vi "Get Wires Info.vi"(11 "connected\nwires refs.":refnum<vi>[](array[refnum])) -> (3 "output cluster 2":T1)   [LabVIEW 2014]
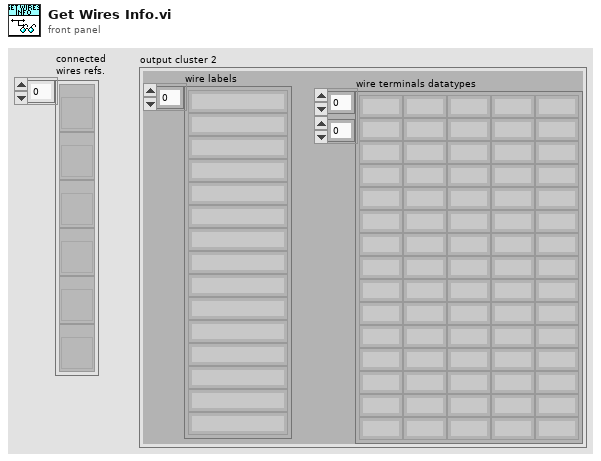
[diagram p1: front panel]
types:
  T1 = cluster{"wire labels":string[], "wire terminals datatypes":string[][]}
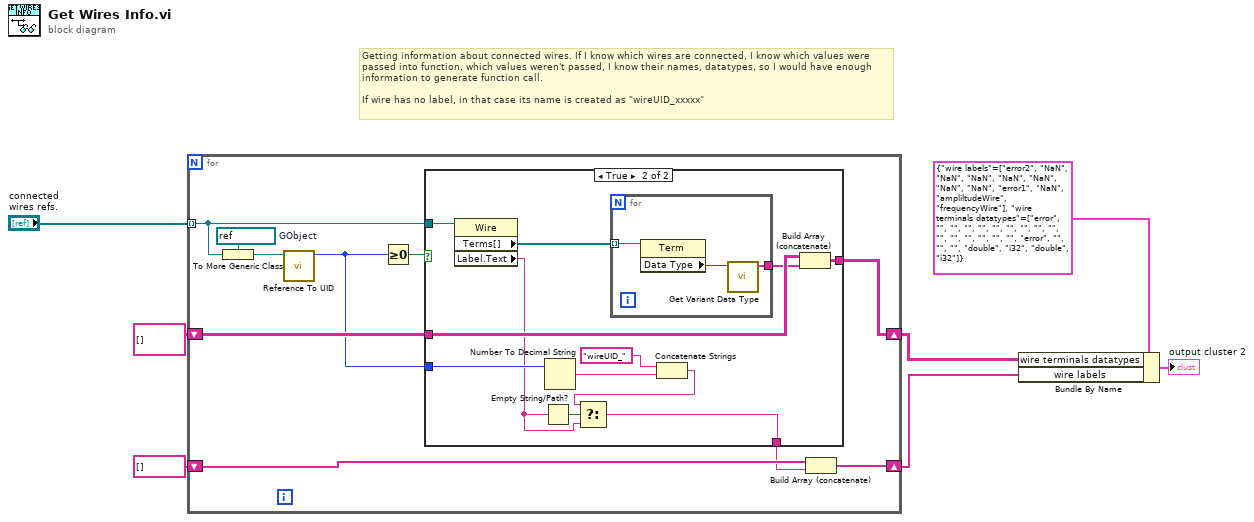
[diagram p0: block diagram]
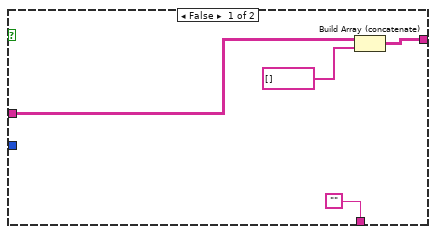
[diagram p2: hidden frame]
diagram:
  # "Getting information about connected wires. If I know which wires are connected, I know which values were passed into function, which values weren't passed, I know their names, datatypes, so I would have enough information to generate function call.\n\nIf wire has no label, in that case its name is created as \"wireUID_xxxxx\""
  n1 = for {
    tunnel: "connected\nwires refs." -> [w9] mode=indexing
    shift-right: [w16] -> w4
    shift-left: string[][] [] -> [w17]
    shift-right: [w11] -> w5
    shift-left: string[] [] -> [w15]
    w8 = refnum<vi> refnum  # GObject
    n2 = To More Generic Class(target class=w8, reference=w9) -> (generic class reference=w10:refnum<vi>)
    n3 = call "Reference To UID.vi"("Reference"=w10) -> ("UID"=w13:i32)  [unwired: 10 in]
    n4 = Greater Or Equal To 0?(x=w13) -> (x >= 0?=w14:bool)
    n5 = case shown="True" w14 {
      tunnel: w9 -> [_ w33]
      tunnel: w17 -> [w19 w32]
      tunnel: [w20 w31] -> w16
      tunnel: ["" w22] -> w12
      tunnel: w13 -> [_ w25]
      frame False {
        n6 = Build Array (concatenate)(w19, string[] [] ("element")) -> (w20:string[][])
      }
      frame True {
        n7 = property class="Wire"(reference=w33) -> ("Terms[]"=w30:refnum<vi>[], "Label.Text"=w23:string)  [unwired: 1 in, 2 out]
        n8 = Empty String/Path?(string/path=w23) -> (empty?=w28:bool)
        n9 = Number To Decimal String(number=w25) -> (decimal integer string=w26:string)  [unwired: 1 in]
        n10 = for {
          tunnel: w30 -> [w36] mode=indexing
          tunnel: [w34] -> w29
          n11 = property class="Term"(reference=w36) -> ("Data Type"=w35:variant)  [unwired: 1 in, 2 out]
          n12 = call "Get Variant Data Type.vi"("variant"=w35) -> ("Data Type"=w34:string[])  [unwired: 10 in]
        }
        n13 = Concatenate Strings("wireUID_" ("string"), w26) -> (w24:string)
        n14 = Select(t=w24, s=w28, f=w23) -> (s? t:f=w22:string)
        n15 = Build Array (concatenate)(w32, w29) -> (w31:string[][])
      }
    }
    n16 = Build Array (concatenate)(w15, w12) -> (w11:string[])
  }
  n17 = Bundle By Name(cluster=T1 {"wire labels"=["error2", "NaN", "NaN", "NaN", "NaN", "NaN", "NaN", "NaN", "error1", "NaN", "ampliltudeWire", "frequencyWire"], "wire terminals datatypes"=[["error", ""], ["", ""], ["", ""], ["", ""], ["", ""], ["", ""], ["", ""], ["", ""], ["error", ""], ["", ""], ["double", "i32"], ["double", "i32"]]}, "wire terminals datatypes"=w4, "wire labels"=w5) -> (→"output cluster 2":T1)
